vi "Mouse Begin.vi"(4 "Timeout (ms)":i32=100, 5 "FPGA VI Reference In":refnum<k20>) -> (0 "Timed out?":bool, 2 "FPGA VI Reference Out":refnum<k20>)   [LabVIEW 2012]
uses:
  <vilib>/Utility/error.llb/Error Cluster From Error Code.vi
  <vilib>/rvi/errors/niLvFpgaAdjustHostInterfaceError.vi
  <vilib>/rvi/interface/nirviReadWriteControl/nirviReadWriteControl.xnode
  NiFpgaLv.dll
  <vilib>/rvi/interface/Simulation/niFpgaSimulationCallBeginRW.vi
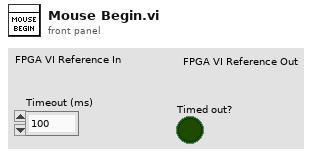
[diagram p1: front panel]
types:
  T1 = enum16{"idle", "set idle", "begin", "write", "read", "power down", "reset"}
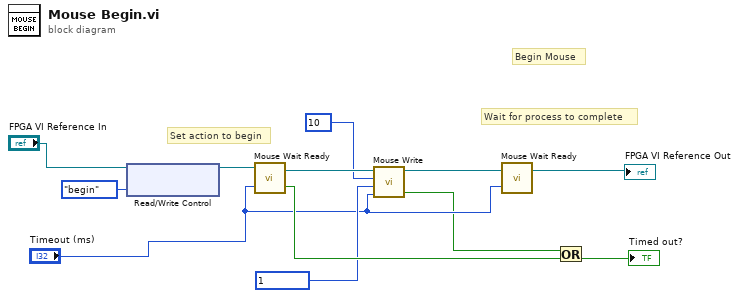
[diagram p0: block diagram]
diagram:
  # "Wait for process to complete"
  # "Set action to begin"
  # "Begin Mouse"
  n1 = xnode "Read/Write Control"("FPGA VI Reference In"="FPGA VI Reference In", "Mouse Action"=T1."begin") -> ("FPGA VI Reference Out"=w11:refnum<k20>)  [unwired: 1 in, 1 out]
  n2 = call "Mouse Wait Ready.vi"("Timeout (ms)"="Timeout (ms)", "Refnum in"=w11) -> ("Timeout"=w8:bool, "Refnum out"=w10:refnum<k20>)
  n3 = call "Mouse Write.vi"("Timeout (ms)"="Timeout (ms)", "Write Data In"=u8 1, "Write Address"=u8 10, "FPGA VI Reference In"=w10) -> ("Timed out?"=w1:bool, "FPGA VI Reference Out"=w7:refnum<k20>)  [unwired: 1 in]
  n4 = call "Mouse Wait Ready.vi"("Timeout (ms)"="Timeout (ms)", "Refnum in"=w7) -> ("Refnum out"=→"FPGA VI Reference Out":refnum<k20>)  [unwired: 1 out]
  n5 = Or(x=w1, y=w8) -> (x .or. y?=→"Timed out?":bool)
